vi "Inject Some Thangs.vi"(8 "error in (no error)":errorcluster, 9 "Attributes Ref":refnum<data-value>, 11 "Popup in":refnum<class "Popup.lvclass">) -> (0 "error out":errorcluster, 3 "Popup out":refnum<class "Popup.lvclass">)   [LabVIEW 2020, in "Test Executive.lvlib" / "Parallelizer Example.lvlib" / "Popup.lvclass"]
uses:
  <vilib>/gpm_packages/@cs/test-executive/Source/Sandbox/Parallelizer Example/Popup/Popup.lvclass
  <vilib>/gpm_packages/@cs/lookup-table/Source/LookupTable/LookupTable.lvclass
  <vilib>/gpm_packages/@cs/lookup-table/Source/LookupTable/LookupTable.lvclass/LookupTable.ctl
  <vilib>/gpm_packages/@cs/test-executive/Source/Sandbox/Parallelizer Example/Popup/Popup.lvclass/Popup.ctl
  42a1093b-6a9b-4c30-b1f5-c056101c5f6c.vi
  <vilib>/gpm_packages/@cs/lookup-table/Source/LookupTable/Read Table Reference.vi
  42a1093b-6a9b-4c30-b1f5-c056101c5f6c.vi/a4e8bcb5-c42e-44e7-90c4-bd809ddd9906.vi
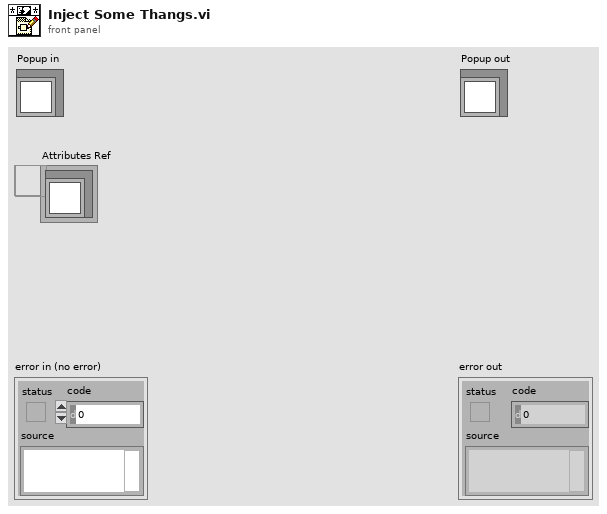
[diagram p1: front panel]
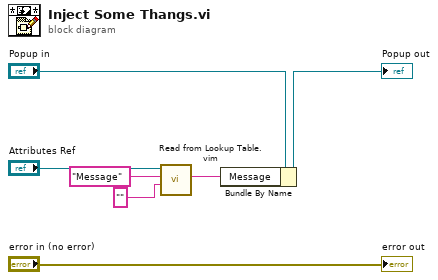
[diagram p0: block diagram]
diagram:
  n1 = call "Read from Lookup Table.vim"("Type"="", "Item Name"="Message", "LookupTable Reference"="Attributes Ref") -> ("Value"=w4:string)  [unwired: 5 in, 3 out]
  n2 = Bundle By Name(cluster="Popup in", "Message"=w4) -> (→"Popup out":refnum<class "Popup.lvclass">)
  "error out" <- "error in (no error)"
